vi "Requests.vi"(8 "error in (no error)":errorcluster, 9 "write enable":bool=TRUE, 11 "ICPCON ET-7017 in":refnum<class "ICPCON PM-3112.lvclass">) -> (0 "error out":errorcluster, 3 "ICPCON ET-7017 out":refnum<class "ICPCON PM-3112.lvclass">)   [LabVIEW 2021, in "ICPCON PM-3112.lvclass"]
uses:
  ICPCON PM-3112.lvclass
  D:/my_projects/projects/Algorithms/Labview/21/Master CR/Master CR.lvclass
  D:/my_projects/projects/Algorithms/Labview/21/Master CR/Devices/ET7000/TCP/TCP.lvclass
  Master CR.lvclass/Master CR.ctl
  Modbus_v121c/Modbus Data Unit/Modbus Data Unit.lvclass/Modbus Data Unit.ctl
  Modbus_v121c/Network Protocol/Network Master/Network Master.lvclass/Network Master.ctl
  Modbus_v121c/Master Function Definition/Read Input Registers Request.vi
  Modbus_v121c/Master Function Definition/Read Input Registers Response.vi
  Modbus_v121c/Network Protocol/Network Master/Read write Master.vi
  Network Protocol/Read Network Protocol.vi
  Modbus_v121c/Modbus Data Unit/Construct PDU.vi
  Modbus_v121c/Utility/Bytes to U16s.vi
  Modbus_v121c/Master Function Definition/Function code mismatch error.vi
  Modbus_v121c/Data Model/Error Generator.vi
  Modbus_v121c/Modbus Data Unit/Deconstruct PDU.vi
  TCP/TCP.lvclass
  Modbus_v121c/Network Protocol/Network Master/Network Master.lvclass
  Modbus_v121c/Modbus Data Unit/Modbus Data Unit.lvclass
  Modbus_v121c/Data Model/Device Data Model.lvclass
  Modbus_v121c/Transmission Data Unit/Transmission Data Unit.lvclass
  Master CR.lvclass
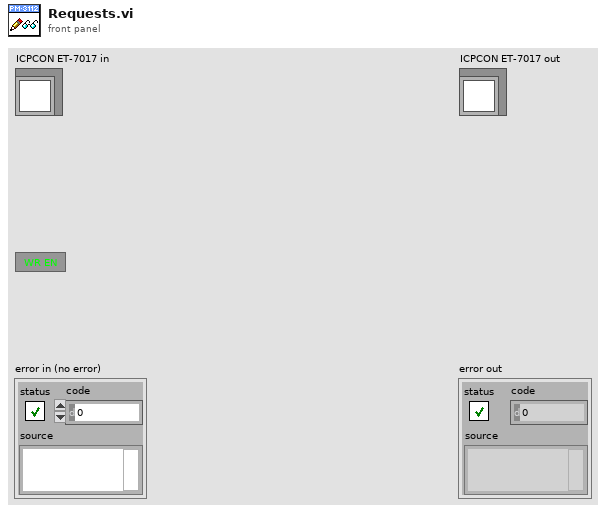
[diagram p1: front panel]
types:
  T1 = typedef "Device Data Model.lvclass/N channel.ctl" = cluster{"N DI channel":i32, "N DO channel":i32, "N AI channel":i32, "N AO channel":i32}
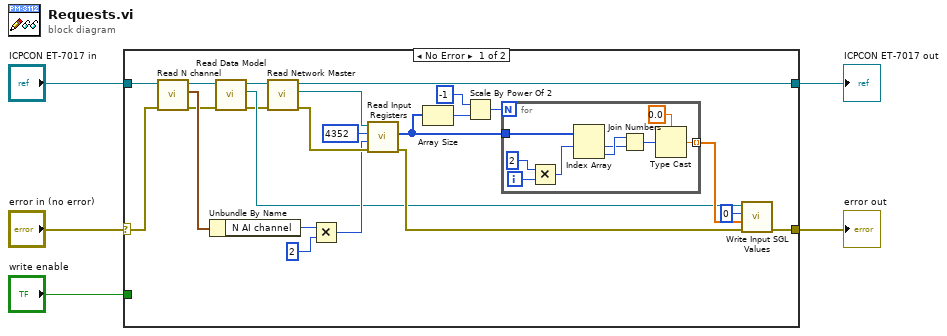
[diagram p0: block diagram]
diagram:
  n1 = case shown="No Error" "error in (no error)" {
    selector: "error in (no error)" -> [w23 w39]
    tunnel: [w20 w39] -> w3
    tunnel: [w16 w38] -> w4
    tunnel: "ICPCON ET-7017 in" -> [w25 w38]
    tunnel: "write enable" -> [_ _]
    frame No Error {
      n2 = call "Read N channel.vi"("error in (no error)"=w23, "Master CR in"=w25) -> ("error out"=w22:errorcluster, "N channel"=w26:T1, "Master CR out"=w24:refnum<class "ICPCON PM-3112.lvclass">)  [unwired: 7 in]
      n3 = Unbundle By Name(w26) -> ("N AI channel"=w14:i32)
      n4 = call "Read Data Model.vi"("error in (no error)"=w22, "Master CR in"=w24) -> ("error out"=w6:errorcluster, "Data Model"=w7:refnum<class "Device Data Model.lvclass">, "Master CR out"=w19:refnum<class "ICPCON PM-3112.lvclass">)  [unwired: 7 in]
      n5 = call "Read Network Master.vi"("error in (no error)"=w6, "TCP in"=w19) -> ("error out"=w17:errorcluster, "Network Master"=w18:refnum<class "Network Master.lvclass">, "TCP out"=w16:refnum<class "ICPCON PM-3112.lvclass">)  [unwired: 7 in]
      n6 = Multiply(x=w14, y=2) -> (x*y=w15:i32)
      n7 = call "Read Input Registers.vi"("error in (no error)"=w17, "number of input registers"=w15, "starting address"=u16 4352, "Modbus master in"=w18) -> ("error out"=w21:errorcluster, "register values"=w9:u16[])  [unwired: 5 in, 1 out]
      n8 = Array Size(array=w9) -> (size(s)=w12:i32)
      n9 = Scale By Power Of 2(n=i16 -1, x=w12) -> (x*2^n=w10:i32)
      n10 = for {
        N: w10 -> [_]
        tunnel: w9 -> [w34]
        tunnel: [w32] -> w8 mode=indexing
        i -> [w37]
        n11 = Multiply(x=2 ("n"), y=w37) -> (x*y=w35:i32)
        n12 = Index Array(array=w34, index #1=w35) -> (element #1=w29:u16, element #2=w30:u16)  [unwired: 1 in]
        n13 = Join Numbers(hi=w30, lo=w29) -> ((hi.lo)=w31:u32)
        n14 = Type Cast(type=sgl 0.0 ("x"), x=w31) -> (*(type *) &x=w32:sgl)
      }
      n15 = call-dynamic "Write Input SGL Values.vi"("error in (no error)"=w21, "values"=w8, "starting address"=u16 0, "standard data model in"=w7) -> ("error out"=w20:errorcluster)  [unwired: 6 in, 1 out]
    }
    frame Error {
    }
  }
  "error out" <- w3
  "ICPCON ET-7017 out" <- w4
